vi "Filters_good_test.vi"() -> ()   [LabVIEW 2009]
uses:
  <vilib>/vision/NI_Vision_Development_Module.lvlib
panel:
  in  "Hough Skip":i32=1
  in  "LineFilterSelect":bool
  out "Hough Intensity Graph":i32[][](graph)
  out "Angle 2":i32
  out "X Intercept 2":i32
  in  "movement_limit":i32
  in  "check_block_size/2":i32
  in  "Waypoint Select":enum32{"Centroid", "Walk", "Mean Hough"}(radio)
  out "AverageTime (s)":dbl
  out "AverageTime (ms)":dbl
  out "ElapsedTime":u32
  out "Waypoint":cluster{i32, i32}
  in  "WP_DisplaySize/2":i32
  out "Filter Binary 2":T1(plugin-control)
  out "Filter Binary":T1(plugin-control)
  in  "file (use dialog)":path=path "C:/Documents and Settings/dgrieneisen/My Documents/Robotics/Athena/weights.fl"
  in  "Stop":bool
  in  "Filter Select":T2(radio)
  out "Filter Settings":T2(tab)
  in  "Red Range":cluster{"Lower value":i32, "Upper value":i32}={"Lower value"=120, "Upper value"=200}
  in  "Green Range":cluster{"Lower value":i32, "Upper value":i32}={"Lower value"=0, "Upper value"=255}
  in  "Blue Range":cluster{"Lower value":i32, "Upper value":i32}={"Lower value"=100, "Upper value"=255}
  in  "Color Mode":u16(ring) items=["RGB", "HSL", "HSV", "HSI"]
  in  "Hue Range":cluster{"Lower value":i32, "Upper value":i32}={"Lower value"=0, "Upper value"=255}
  in  "Saturation Range":cluster{"Lower value":i32, "Upper value":i32}={"Lower value"=0, "Upper value"=255}
  in  "Luma Range":cluster{"Lower value":i32, "Upper value":i32}={"Lower value"=0, "Upper value"=255}
  in  "Color Mode HSL":u16(ring)=1 items=["RGB", "HSL", "HSV", "HSI"]
  in  "Red Scalar":sgl=3.0
  in  "Green Scalar":sgl=3.0
  in  "Blue Scalar":sgl=3.3
  in  "Luma Scalar Low":sgl=4.0
  in  "Sat Scalar":sgl=2.5
  in  "Hue Scalar":sgl=5.0
  in  "Luma Scalar High":sgl=4.0
  in  "res/2":i32=3
  in  "Sample Rate":i32=3
  in  "ANN Level":dbl=0.5
  in  "ANN Out Switch":bool
  in  "Input Image Path":path=path "C:/Documents and Settings/dgrieneisen/My Documents/Robotics/Athena/image2004.jpg"
  out "'input Image":T1(plugin-control)
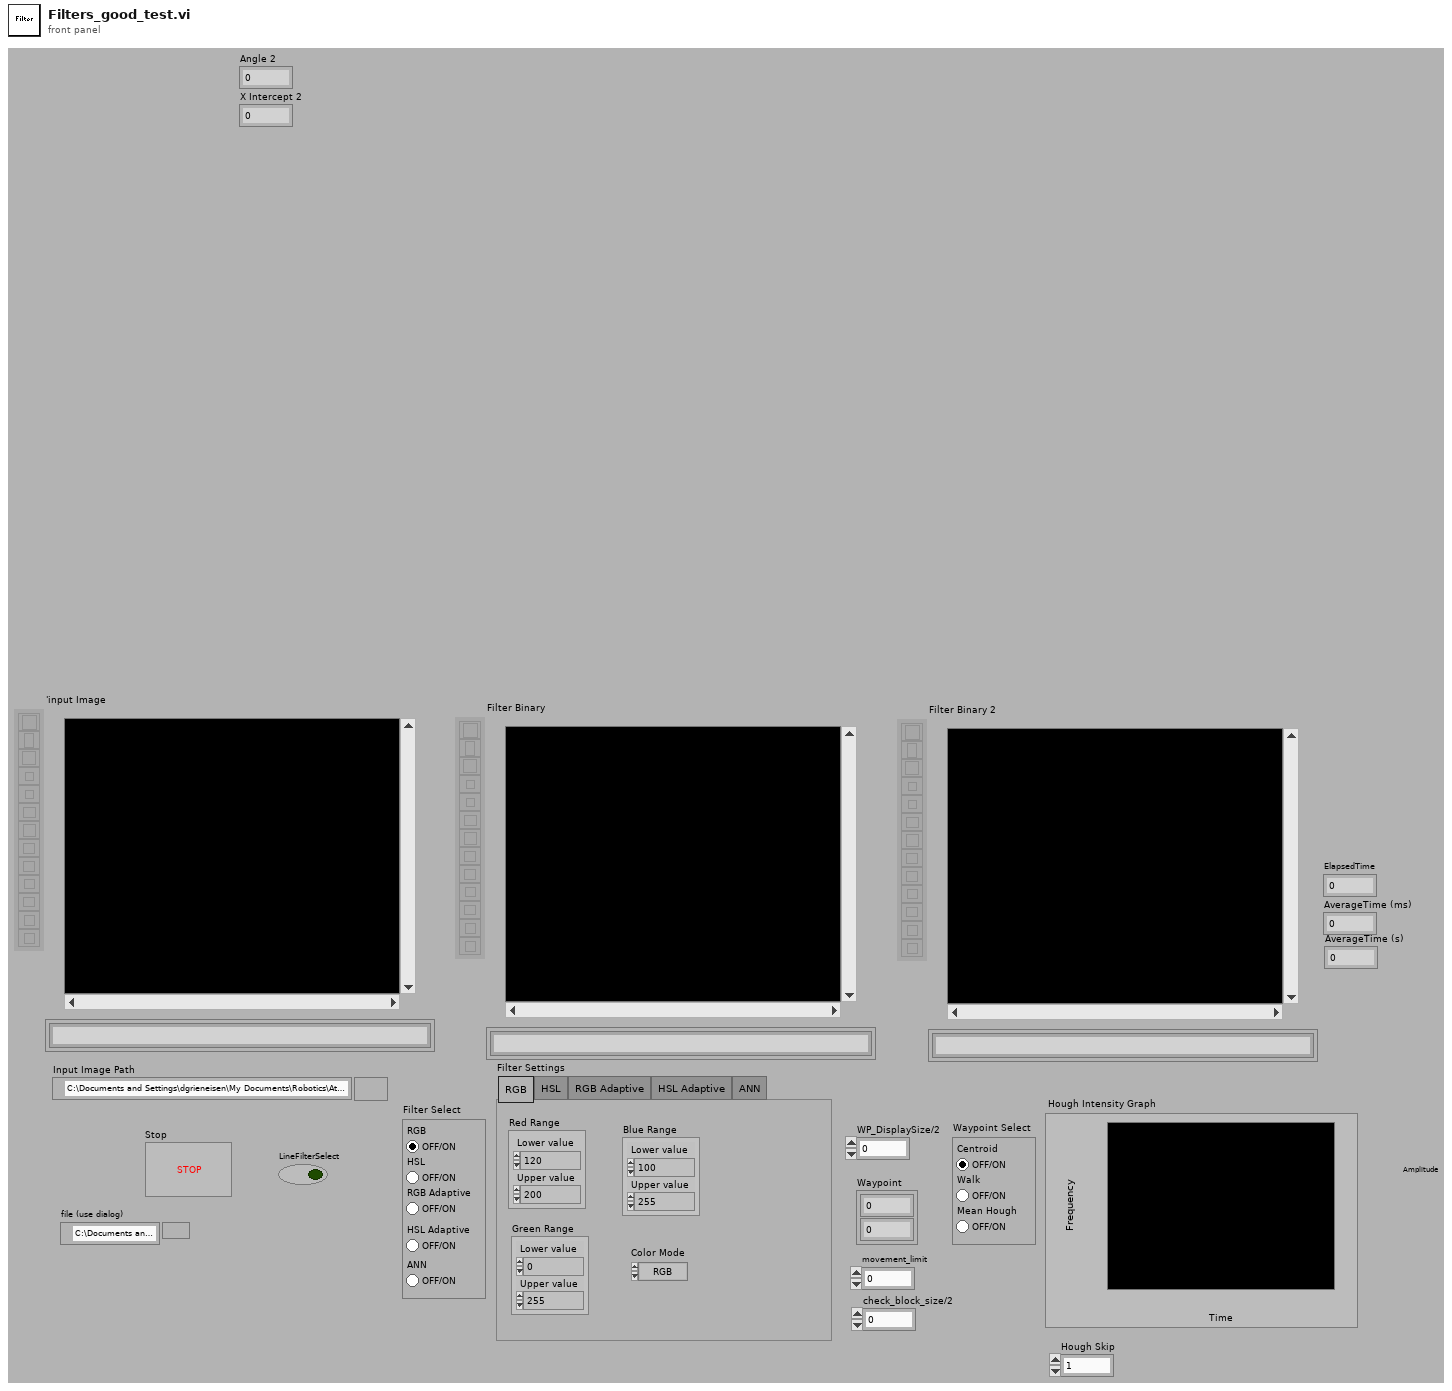
[diagram p1: front panel]
types:
  T1 = typedef "IMAQ Image.ctl" = refnum<image>
  T2 = enum32{"RGB", "HSL", "RGB Adaptive", "HSL Adaptive", "ANN"}
  T3 = typedef "Image Type" = u32
  T4 = cluster{"Num Hidden Layer":i32, "Function Final Layer":u16, "Function Hidden Layer":u16, dbl[], dbl[][]}
  T5 = cluster{"Left":i32, "Top":i32, "Right":i32, "Bottom":i32}
  T6 = cluster{"histogram":u32[], "Minimal Value":sgl, "Maximal Value":sgl, "Starting Value":sgl, "Interval Width":sgl, "Mean Value":sgl, "Standard  Variation":sgl, "Area (pixels)":i32}
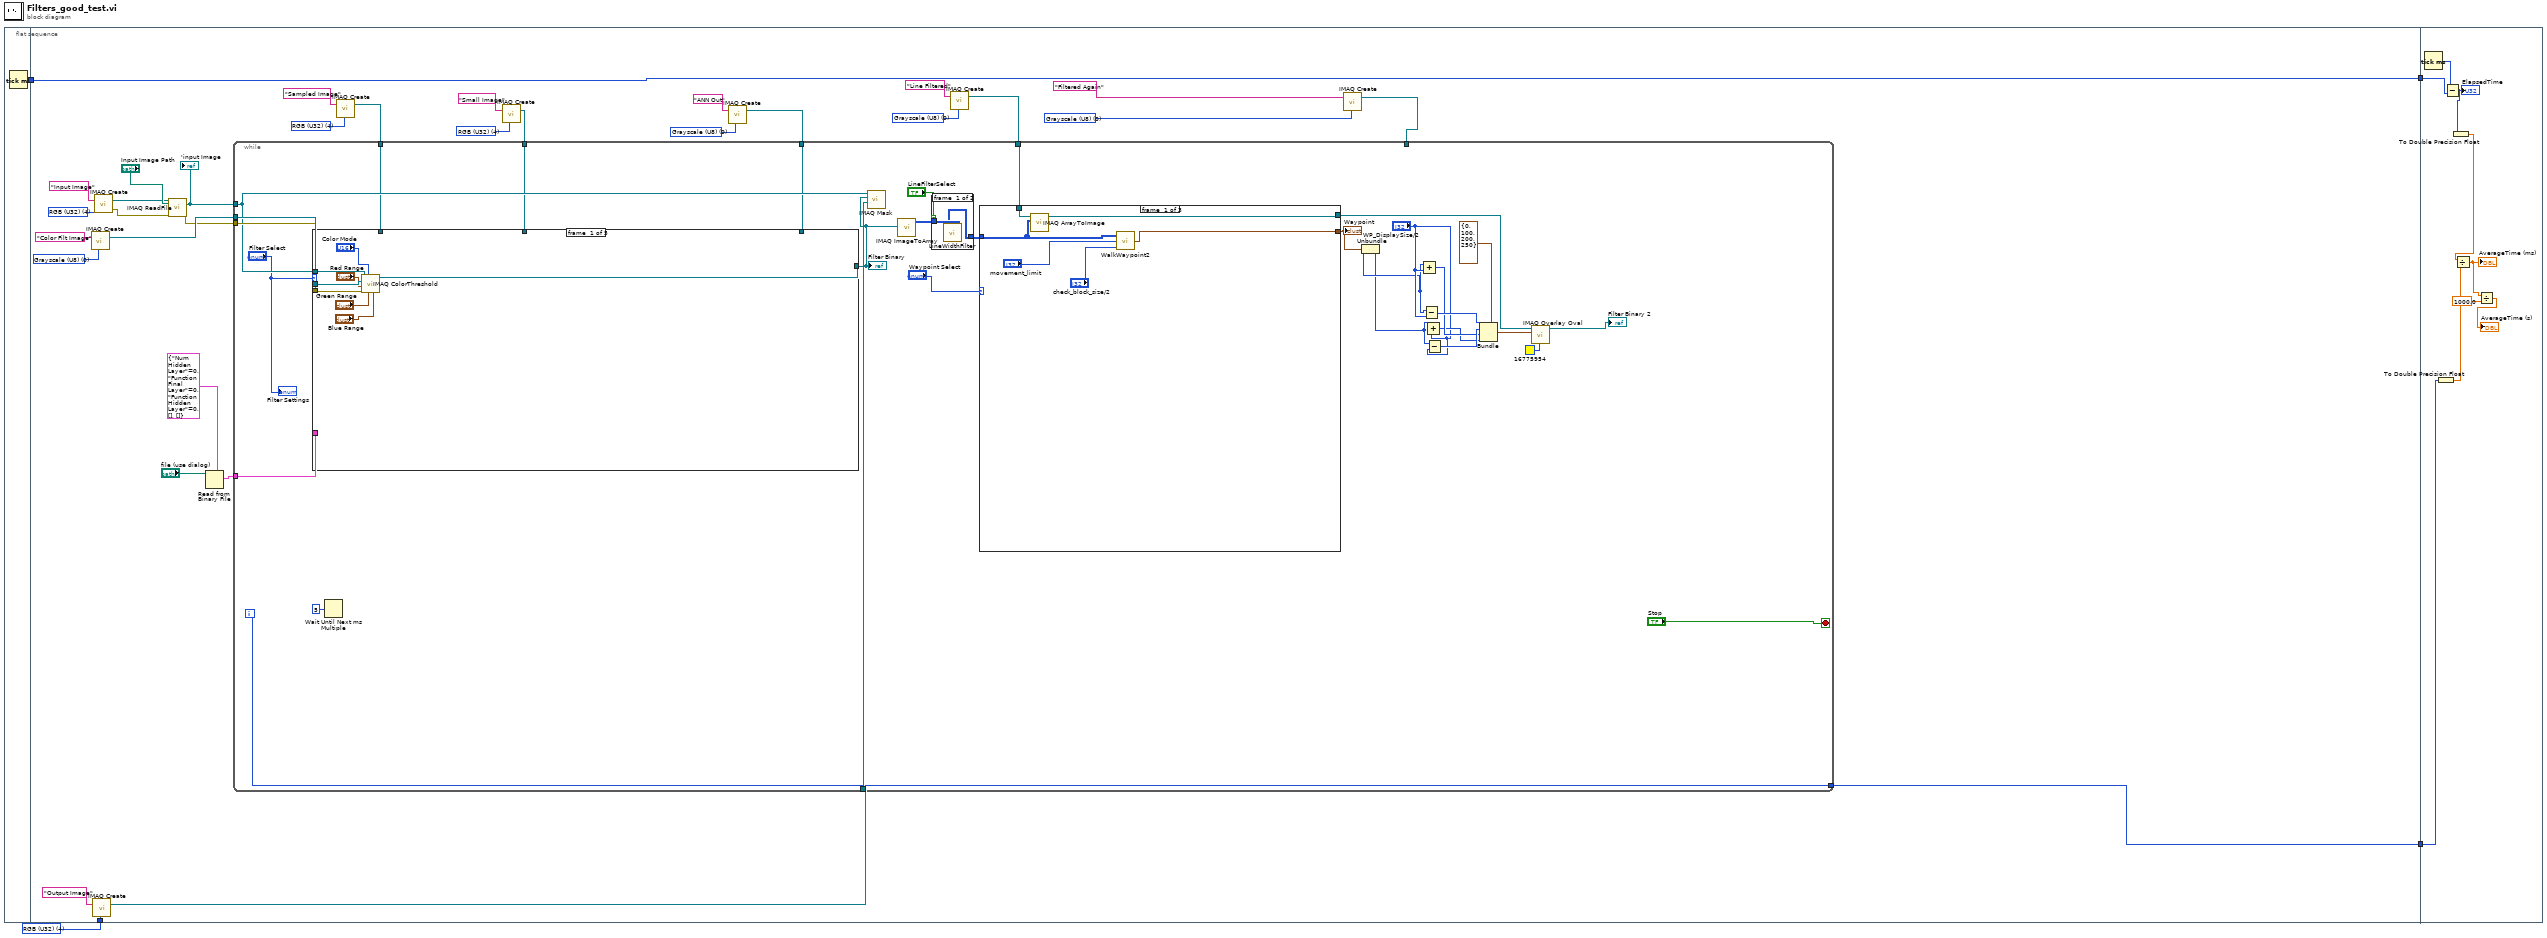
[diagram p0: block diagram]
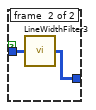
[diagram p2: hidden frame]
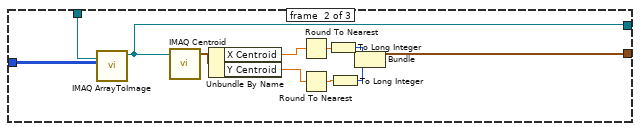
[diagram p3: hidden frame]
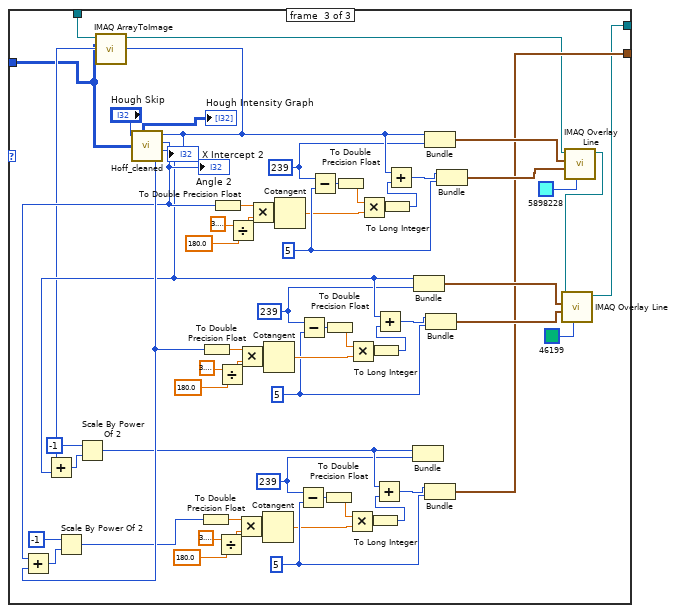
[diagram p4: hidden frame]
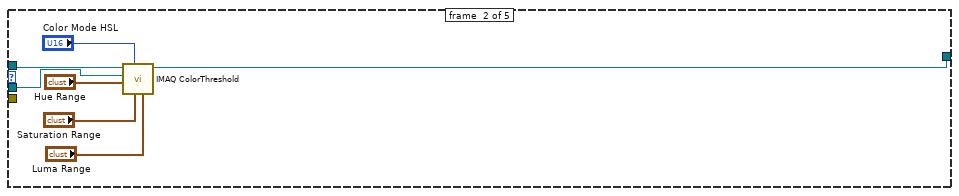
[diagram p5: hidden frame]
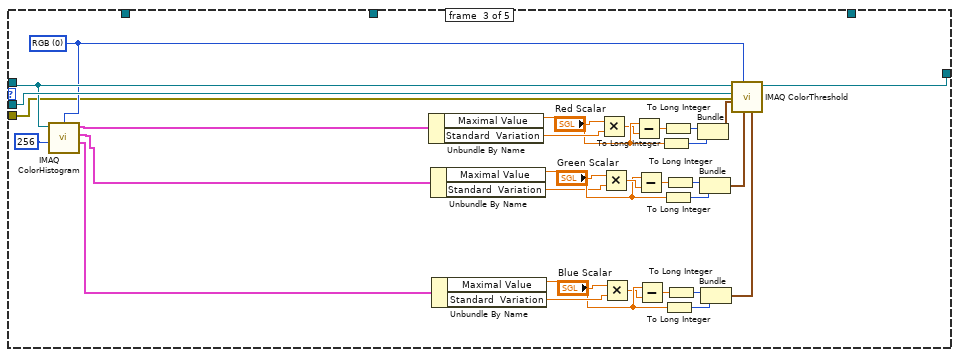
[diagram p6: hidden frame]
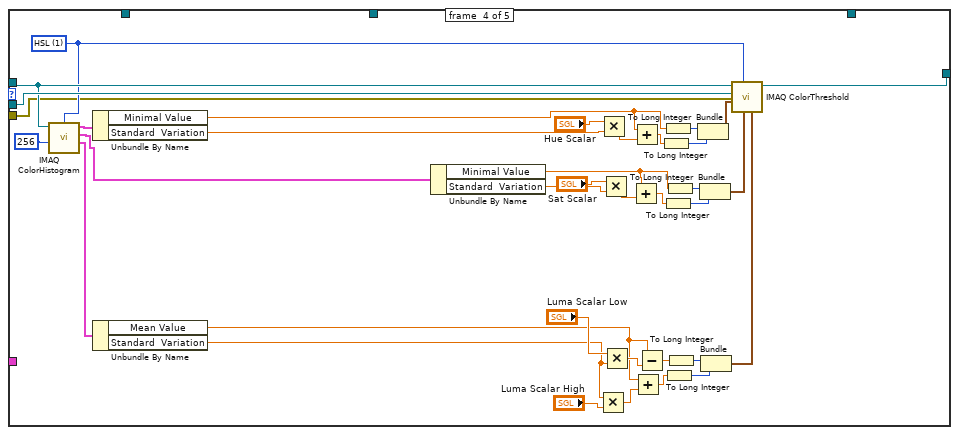
[diagram p7: hidden frame]
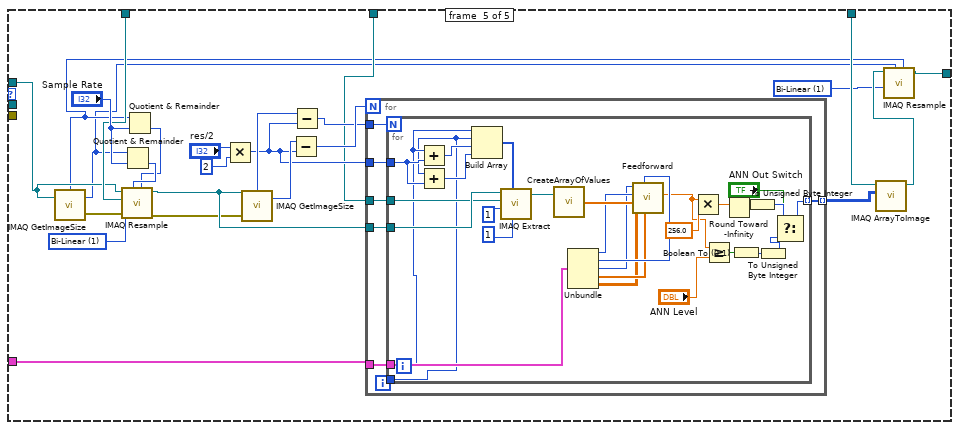
[diagram p8: hidden frame]
diagram:
  w4 = T3 4 items=["Grayscale (U8)", "Grayscale (I16)", "Grayscale (SGL)", "Complex (CSG)", "RGB (U32)", "HSL (U32)", "RGB (U64)", "Grayscale (U16)"] ("Image Type")
  n1 = flat-sequence {
    tunnel: [w5] -> w3
    tunnel: w4 -> [w34]
    tunnel: w3 -> [w8]
    tunnel: [w8] -> w2
    tunnel: [w7] -> w1
    tunnel: w2 -> [w306]
    tunnel: w1 -> [w305]
    frame #0 {
      n2 = Tick Count (ms)() -> (millisecond timer value=w5:u32)
    }
    frame #1 {
      w11 = T3 0 items=["Grayscale (U8)", "Grayscale (I16)", "Grayscale (SGL)", "Complex (CSG)", "RGB (U32)", "HSL (U32)", "RGB (U64)", "Grayscale (U16)"] ("Image Type")
      w12 = T3 0 items=["Grayscale (U8)", "Grayscale (I16)", "Grayscale (SGL)", "Complex (CSG)", "RGB (U32)", "HSL (U32)", "RGB (U64)", "Grayscale (U16)"] ("Image Type")
      w17 = T3 0 items=["Grayscale (U8)", "Grayscale (I16)", "Grayscale (SGL)", "Complex (CSG)", "RGB (U32)", "HSL (U32)", "RGB (U64)", "Grayscale (U16)"] ("Image Type")
      w21 = T3 4 items=["Grayscale (U8)", "Grayscale (I16)", "Grayscale (SGL)", "Complex (CSG)", "RGB (U32)", "HSL (U32)", "RGB (U64)", "Grayscale (U16)"] ("Image Type")
      w25 = T3 4 items=["Grayscale (U8)", "Grayscale (I16)", "Grayscale (SGL)", "Complex (CSG)", "RGB (U32)", "HSL (U32)", "RGB (U64)", "Grayscale (U16)"] ("Image Type")
      w36 = T3 0 items=["Grayscale (U8)", "Grayscale (I16)", "Grayscale (SGL)", "Complex (CSG)", "RGB (U32)", "HSL (U32)", "RGB (U64)", "Grayscale (U16)"] ("Image Type")
      w38 = T3 4 items=["Grayscale (U8)", "Grayscale (I16)", "Grayscale (SGL)", "Complex (CSG)", "RGB (U32)", "HSL (U32)", "RGB (U64)", "Grayscale (U16)"] ("Image Type")
      n3 = call "IMAQ Create"("Image Name"="Color Filt Image", "Image Type"=w36) -> ("New Image"=w30:T1)  [unwired: 2 in, 2 out]
      n4 = call "IMAQ Create"("Image Name"="Output Image", "Image Type"=w34) -> ("New Image"=w28:T1)  [unwired: 2 in, 2 out]
      n5 = call "IMAQ Create"("Image Name"="Input Image", "Image Type"=w38) -> ("New Image"=w27:T1, "error out"=w31:errorcluster)  [unwired: 2 in, 1 out]
      n6 = call "IMAQ ReadFile"("File Path"="Input Image Path", "error in (no error)"=w31, "Image"=w27) -> ("error out"=w29:errorcluster, "Image Out"=w26:T1)  [unwired: 4 in, 3 out]
      "'input Image" <- w26
      n7 = Read from Binary File(5:T4 {"Num Hidden Layer"=0, "Function Final Layer"=0, "Function Hidden Layer"=0, [], []} ("Cluster"), 11:"file (use dialog)") -> (2:w19:T4)  [unwired: 4 in, 3 out]
      n8 = call "IMAQ Create"("Image Name"="Sampled Image", "Image Type"=w25) -> ("New Image"=w23:T1)  [unwired: 2 in, 2 out]
      n9 = call "IMAQ Create"("Image Name"="Small Image", "Image Type"=w21) -> ("New Image"=w20:T1)  [unwired: 2 in, 2 out]
      n10 = call "IMAQ Create"("Image Name"="ANN Out", "Image Type"=w17) -> ("New Image"=w15:T1)  [unwired: 2 in, 2 out]
      n11 = call "IMAQ Create"("Image Name"="Line Filtered", "Image Type"=w12) -> ("New Image"=w6:T1)  [unwired: 2 in, 2 out]
      n12 = call "IMAQ Create"("Image Name"="Filtered Again", "Image Type"=w11) -> ("New Image"=w9:T1)  [unwired: 2 in, 2 out]
      n13 = while {
        tunnel: w30 -> [w69]
        tunnel: w29 -> [w68]
        tunnel: w28 -> [w67]
        tunnel: w26 -> [w66]
        tunnel: w23 -> [w63]
        tunnel: w20 -> [w62]
        tunnel: w19 -> [w61]
        tunnel: w15 -> [w60]
        tunnel: w6 -> [w57]
        tunnel: w9 -> [_]
        tunnel: [w48] -> w7
        i -> [w48]
        stop <- "Stop" stop-if-true
        n14 = case shown="\"ANN\"" "Filter Select" {
          tunnel: w69 -> [w161 w166 w200 w236 _]
          tunnel: w68 -> [w160 _ w187 w226 _]
          tunnel: w66 -> [w156 w167 w199 w235 w246]
          tunnel: [w154 w162 w201 w237 w241] -> w59
          tunnel: w63 -> [_ _ _ _ w247]
          tunnel: w62 -> [_ _ _ _ w245]
          tunnel: w61 -> [_ _ _ _ w244]
          tunnel: w60 -> [_ _ _ _ w243]
          frame #0 {
            n15 = call "IMAQ ColorThreshold"("Blue or Luma or Val or Inten Range"="Blue Range", "Green or Sat Range"="Green Range", "Color Mode"="Color Mode", "error in (no error)"=w160, "Red or Hue Range"="Red Range", "Image Dst"=w161, "Image Src"=w156) -> ("Image Dst Out"=w154:T1)  [unwired: 3 in, 1 out]
          }
          frame #1 {
            n16 = call "IMAQ ColorThreshold"("Blue or Luma or Val or Inten Range"="Luma Range", "Green or Sat Range"="Saturation Range", "Color Mode"="Color Mode HSL", "Red or Hue Range"="Hue Range", "Image Dst"=w166, "Image Src"=w167) -> ("Image Dst Out"=w162:T1)  [unwired: 4 in, 1 out]
          }
          frame #2 {
            w197 = u16 0 items=["RGB", "HSL", "HSV", "HSI"] ("Color Mode")
            n17 = call "IMAQ ColorHistogram"("Color Mode"=w197, "Image Src"=w199, "Number of Classes"=256) -> ("Red or Hue or X or L* Histogram Report"=w196:T6, "Green or Sat or Y or a* Histogram Report"=w170:T6, "Blue or Luma or Val or Inten or Z or b* Histogram Report"=w169:T6)  [unwired: 3 in, 1 out]
            n18 = Unbundle By Name(w196) -> ("Maximal Value"=w190:sgl, "Standard  Variation"=w192:sgl)
            n19 = Unbundle By Name(w170) -> ("Maximal Value"=w184:sgl, "Standard  Variation"=w182:sgl)
            n20 = Unbundle By Name(w169) -> ("Maximal Value"=w175:sgl, "Standard  Variation"=w177:sgl)
            n21 = Multiply(x="Red Scalar", y=w192) -> (x*y=w189:sgl)
            n22 = Multiply(x="Green Scalar", y=w182) -> (x*y=w185:sgl)
            n23 = Multiply(x="Blue Scalar", y=w177) -> (x*y=w174:sgl)
            n24 = Subtract(x=w190, y=w189) -> (x-y=w191:sgl)
            n25 = Subtract(x=w184, y=w185) -> (x-y=w183:sgl)
            n26 = Subtract(x=w175, y=w174) -> (x-y=w176:sgl)
            n27 = To Long Integer(number=w190) -> (32bit integer=w193:i32)
            n28 = To Long Integer(number=w191) -> (32bit integer=w194:i32)
            n29 = To Long Integer(number=w184) -> (32bit integer=w181:i32)
            n30 = To Long Integer(number=w175) -> (32bit integer=w178:i32)
            n31 = To Long Integer(number=w183) -> (32bit integer=w180:i32)
            n32 = To Long Integer(number=w176) -> (32bit integer=w179:i32)
            n33 = Bundle(w194, w193) -> (w195:cluster{i32, i32})  [unwired: 1 in]
            n34 = Bundle(w180, w181) -> (w172:cluster{i32, i32})  [unwired: 1 in]
            n35 = Bundle(w179, w178) -> (w171:cluster{i32, i32})  [unwired: 1 in]
            n36 = call "IMAQ ColorThreshold"("Blue or Luma or Val or Inten Range"=w171, "Green or Sat Range"=w172, "Color Mode"=w197, "error in (no error)"=w187, "Red or Hue Range"=w195, "Image Dst"=w200, "Image Src"=w199) -> ("Image Dst Out"=w201:T1)  [unwired: 3 in, 1 out]
          }
          frame #3 {
            w233 = u16 1 items=["RGB", "HSL", "HSV", "HSI"] ("Color Mode")
            n37 = call "IMAQ ColorHistogram"("Color Mode"=w233, "Image Src"=w235, "Number of Classes"=256) -> ("Red or Hue or X or L* Histogram Report"=w232:T6, "Green or Sat or Y or a* Histogram Report"=w216:T6, "Blue or Luma or Val or Inten or Z or b* Histogram Report"=w215:T6)  [unwired: 3 in, 1 out]
            n38 = Unbundle By Name(w232) -> ("Minimal Value"=w213:sgl, "Standard  Variation"=w228:sgl)
            n39 = Unbundle By Name(w215) -> ("Mean Value"=w203:sgl, "Standard  Variation"=w206:sgl)
            n40 = Unbundle By Name(w216) -> ("Minimal Value"=w211:sgl, "Standard  Variation"=w224:sgl)
            n41 = Multiply(x=w206, y="Luma Scalar High") -> (x*y=w204:sgl)
            n42 = Multiply(x="Hue Scalar", y=w228) -> (x*y=w214:sgl)
            n43 = Multiply(x="Sat Scalar", y=w224) -> (x*y=w210:sgl)
            n44 = Multiply(x="Luma Scalar Low", y=w206) -> (x*y=w219:sgl)
            n45 = Add(x=w211, y=w210) -> (x+y=w209:sgl)
            n46 = Add(x=w213, y=w214) -> (x+y=w212:sgl)
            n47 = Add(x=w203, y=w204) -> (x+y=w205:sgl)
            n48 = Subtract(x=w203, y=w219) -> (x-y=w220:sgl)
            n49 = To Long Integer(number=w212) -> (32bit integer=w229:i32)
            n50 = To Long Integer(number=w213) -> (32bit integer=w230:i32)
            n51 = To Long Integer(number=w209) -> (32bit integer=w223:i32)
            n52 = To Long Integer(number=w205) -> (32bit integer=w202:i32)
            n53 = To Long Integer(number=w211) -> (32bit integer=w222:i32)
            n54 = To Long Integer(number=w220) -> (32bit integer=w221:i32)
            n55 = Bundle(w230, w229) -> (w231:cluster{i32, i32})  [unwired: 1 in]
            n56 = Bundle(w222, w223) -> (w218:cluster{i32, i32})  [unwired: 1 in]
            n57 = Bundle(w221, w202) -> (w217:cluster{i32, i32})  [unwired: 1 in]
            n58 = call "IMAQ ColorThreshold"("Blue or Luma or Val or Inten Range"=w217, "Green or Sat Range"=w218, "Color Mode"=w233, "error in (no error)"=w226, "Red or Hue Range"=w231, "Image Dst"=w236, "Image Src"=w235) -> ("Image Dst Out"=w237:T1)  [unwired: 3 in, 1 out]
          }
          frame #4 {
            w240 = u32 1 items=["Zero Order", "Bi-Linear", "Quadratic", "Cubic Spline"] ("Interpolation Type")
            w258 = u32 1 items=["Zero Order", "Bi-Linear", "Quadratic", "Cubic Spline"] ("Interpolation Type")
            n59 = call "IMAQ GetImageSize"("Image"=w246) -> ("Y Resolution"=w238:i32, "X Resolution"=w239:i32, "error out"=w262:errorcluster)  [unwired: 3 in]
            n60 = Quotient & Remainder(x=w238, y="Sample Rate") -> (floor(x/y)=w261:i32)  [unwired: 1 out]
            n61 = Quotient & Remainder(x=w239, y="Sample Rate") -> (floor(x/y)=w260:i32)  [unwired: 1 out]
            n62 = call "IMAQ Resample"("X Resolution"=w260, "Y Resolution"=w261, "error in (no error)"=w262, "Interpolation Type"=w258, "Image Dst"=w247, "Image Src"=w246) -> ("error out"=w248:errorcluster, "Image Dst Out"=w252:T1)  [unwired: 4 in]
            n63 = Multiply(x="res/2", y=2) -> (x*y=w253:i32)
            n64 = call "IMAQ GetImageSize"("Image"=w252, "error in (no error)"=w248) -> ("Y Resolution"=w257:i32, "X Resolution"=w254:i32)  [unwired: 2 in, 1 out]
            n65 = Subtract(x=w257, y=w253) -> (x-y=w250:i32)
            n66 = Subtract(x=w254, y=w253) -> (x-y=w249:i32)
            n67 = for {
              N: w250 -> [_]
              tunnel: w253 -> [w269]
              tunnel: w252 -> [w268]
              tunnel: w244 -> [w267]
              tunnel: [w266] -> w251 mode=indexing
              tunnel: w245 -> [w265]
              tunnel: w249 -> [w264]
              i -> [w263]
              n68 = for {
                N: w264 -> [_]
                tunnel: w269 -> [w295]
                tunnel: w268 -> [w293]
                tunnel: w267 -> [w290]
                tunnel: [w271] -> w266 mode=indexing
                tunnel: w265 -> [w284]
                tunnel: w263 -> [w280]
                i -> [w281]
                n69 = Add(x=w281, y=w295) -> (x+y=w297:i32)
                n70 = Add(x=w280, y=w295) -> (x+y=w296:i32)
                n71 = Build Array(w281, w280, w297, w296) -> (w294:i32[])
                n72 = call "IMAQ Extract"("Y Step Size"=1, "Optional Rectangle"=w294, "X Step Size"=1, "Image Dst"=w284, "Image Src"=w293) -> ("Image Dst Out"=w292:T1)  [unwired: 1 in, 5 out]
                n73 = call "CreateArrayOfValues.vi"("Image Out"=w292) -> ("Array"=w291:dbl[])  [unwired: 1 in]
                n74 = Unbundle(w290) -> ("Num Hidden Layer"=w289:i32, "Function Final Layer"=w288:u16, "Function Hidden Layer"=w287:u16, w286:dbl[], w285:dbl[][])
                n75 = call "Feedforward.vi"("Final Weights"=w286, "Function Final Layer"=w288, "Hidden Weights"=w285, "Inputs"=w291, "Num Hidden Layer"=w289, "Function Hidden Layer"=w287) -> ("Output"=w276:dbl)  [unwired: 3 out]
                n76 = Multiply(x=w276, y=256.0) -> (x*y=w282:dbl)
                n77 = Greater Or Equal?(x=w276, y="ANN Level") -> (x >= y?=w278:bool)
                n78 = Round Toward -Infinity(1:w282) -> (0:w275:dbl)
                n79 = Boolean To (0,1)(Boolean=w278) -> (0, 1=w274:i16)
                n80 = To Unsigned Byte Integer(number=w275) -> (unsigned 8bit integer=w272:u8)
                n81 = To Unsigned Byte Integer(number=w274) -> (unsigned 8bit integer=w273:u8)
                n82 = Select(t=w272, s="ANN Out Switch", f=w273) -> (s? t:f=w271:u8)
              }
            }
            n83 = call "IMAQ ArrayToImage"("Image Pixels (U8)"=w251, "Image"=w243) -> ("Image Out"=w242:T1)  [unwired: 8 in, 1 out]
            n84 = call "IMAQ Resample"("X Resolution"=w239, "Y Resolution"=w238, "Interpolation Type"=w240, "Image Src"=w242) -> ("Image Dst Out"=w241:T1)  [unwired: 6 in, 1 out]
          }
        }
        "Filter Binary" <- w59
        n85 = Wait Until Next ms Multiple(millisecond multiple=u32 5) -> ()  [unwired: 1 out]
        n86 = call "IMAQ Mask"("Image Dst"=w67, "Image Mask"=w59, "Image Src"=w66) -> ()  [unwired: 2 in, 2 out]
        n87 = call "IMAQ ImageToArray"("Image"=w59) -> ("Image Pixels (U8)"=w58:u8[][])  [unwired: 3 in, 4 out]
        n88 = case shown="False" "LineFilterSelect" {
          tunnel: w58 -> [w71 w73]
          tunnel: [w70 w72] -> w40
          frame #0 {
            n89 = call "LineWidthFilter.vi"("Image Pixels (U8) 2"=w71) -> ("Image Pixels (U8)"=w70:u8[][])
          }
          frame #1 {
            n90 = call "LineWidthFilter3.vi"("Image Pixels (U8) 2"=w73) -> ("Image Pixels (U8)"=w72:u8[][])
          }
        }
        n91 = case shown="\"Mean Hough\"" "Waypoint Select" {
          tunnel: w57 -> [w76 w90 w94]
          tunnel: [w77 w80 w96] -> w43
          tunnel: w40 -> [w75 w89 w95]
          tunnel: [w74 w88 w92] -> w47
          frame #0 {
            n92 = call "IMAQ ArrayToImage"("Image Pixels (U8)"=w75, "Image"=w76) -> ("Image Out"=w74:T1)  [unwired: 8 in, 1 out]
            n93 = call "WalkWaypoint2.vi"("check_block_size/2"="check_block_size/2", "movement_limit"="movement_limit", "Image Pixels (U8)"=w75) -> ("WaypointOut"=w77:cluster{i32, i32})
          }
          frame #1 {
            n94 = call "IMAQ ArrayToImage"("Image Pixels (U8)"=w89, "Image"=w90) -> ("Image Out"=w88:T1)  [unwired: 8 in, 1 out]
            n95 = call "IMAQ Centroid"("Image"=w88) -> ("Centroid"=w87:cluster{"X Centroid":sgl, "Y Centroid":sgl})  [unwired: 3 in, 1 out]
            n96 = Unbundle By Name(w87) -> ("X Centroid"=w84:sgl, "Y Centroid"=w83:sgl)
            n97 = Round To Nearest(number=w84) -> (nearest integer value=w86:sgl)
            n98 = Round To Nearest(number=w83) -> (nearest integer value=w85:sgl)
            n99 = To Long Integer(number=w86) -> (32bit integer=w82:i32)
            n100 = To Long Integer(number=w85) -> (32bit integer=w81:i32)
            n101 = Bundle(w82, w81) -> (w80:cluster{i32, i32})  [unwired: 1 in]
          }
          frame #2 {
            w139 = 5 ("y")
            w138 = 239 ("y")
            w117 = 5 ("y")
            w118 = 239 ("y")
            w106 = 5 ("y")
            w105 = 239 ("y")
            n102 = call "IMAQ ArrayToImage"("Image Pixels (U8)"=w95, "Image"=w94) -> ("Image Out"=w93:T1)  [unwired: 8 in, 1 out]
            n103 = call "Hoff_cleaned.vi"("Skip-1"="Hough Skip", "Image Pixels (U8)"=w95) -> ("3 times averaged"=→"Hough Intensity Graph":i32[][], "X Intercept"=w150:i32, "Angle"=w152:i32, "X Intercept 2"=w151:i32, "Angle 2"=w153:i32)  [unwired: 2 in]
            "Angle 2" <- w152
            "X Intercept 2" <- w150
            n104 = Add(x=w152, y=w153) -> (x+y=w149:i32)
            n105 = Add(x=w150, y=w151) -> (x+y=w148:i32)
            n106 = Scale By Power Of 2(n=i16 -1, x=w149) -> (x*2^n=w145:i32)
            n107 = Scale By Power Of 2(n=i16 -1, x=w148) -> (x*2^n=w147:i32)
            n108 = To Double Precision Float(number=w145) -> (double precision float=w133:dbl)
            n109 = To Double Precision Float(number=w153) -> (double precision float=w123:dbl)
            n110 = To Double Precision Float(number=w152) -> (double precision float=w100:dbl)
            n111 = Divide(x=3.141592653589793, y=180.0) -> (x/y=w134:dbl)
            n112 = Divide(x=3.141592653589793, y=180.0) -> (x/y=w122:dbl)
            n113 = Divide(x=3.141592653589793, y=180.0) -> (x/y=w101:dbl)
            n114 = Multiply(x=w133, y=w134) -> (x*y=w135:dbl)
            n115 = Multiply(x=w123, y=w122) -> (x*y=w121:dbl)
            n116 = Multiply(x=w100, y=w101) -> (x*y=w102:dbl)
            n117 = Cotangent(1:w135) -> (0:w136:dbl)
            n118 = Cotangent(1:w121) -> (0:w120:dbl)
            n119 = Cotangent(1:w102) -> (0:w103:dbl)
            n120 = Subtract(x=w138, y=w139) -> (x-y=w140:i32)
            n121 = Subtract(x=w118, y=w117) -> (x-y=w116:i32)
            n122 = Subtract(x=w105, y=w106) -> (x-y=w109:i32)
            n123 = To Double Precision Float(number=w140) -> (double precision float=w141:dbl)
            n124 = To Double Precision Float(number=w116) -> (double precision float=w115:dbl)
            n125 = To Double Precision Float(number=w109) -> (double precision float=w110:dbl)
            n126 = Multiply(x=w141, y=w136) -> (x*y=w142:dbl)
            n127 = Multiply(x=w115, y=w120) -> (x*y=w114:dbl)
            n128 = Multiply(x=w110, y=w103) -> (x*y=w111:dbl)
            n129 = To Long Integer(number=w142) -> (32bit integer=w143:i32)
            n130 = To Long Integer(number=w114) -> (32bit integer=w113:i32)
            n131 = Add(x=w147, y=w143) -> (x+y=w137:i32)
            n132 = Add(x=w151, y=w113) -> (x+y=w119:i32)
            n133 = To Long Integer(number=w111) -> (32bit integer=w112:i32)
            n134 = Add(x=w150, y=w112) -> (x+y=w104:i32)
            n135 = Bundle(w147, "y"=w138) -> ()  [unwired: 1 in, 1 out]
            n136 = Bundle("X Intercept 2"=w151, "y"=w118) -> (w128:cluster{"X Intercept 2":i32, "y":i32})  [unwired: 1 in]
            n137 = Bundle("X Intercept"=w150, "y"=w105) -> (w107:cluster{"X Intercept":i32, "y":i32})  [unwired: 1 in]
            n138 = Bundle(w137, "y"=w139) -> (w96:cluster{i32, "y":i32})  [unwired: 1 in]
            n139 = Bundle(w119, "y"=w117) -> (w129:cluster{i32, "y":i32})  [unwired: 1 in]
            n140 = Bundle(w104, "y"=w106) -> (w108:cluster{i32, "y":i32})  [unwired: 1 in]
            n141 = call "IMAQ Overlay Line"("Color"=u32 5898228, "End Point"=w108, "Start Point"=w107, "Image"=w93) -> ("Image Out"=w130:T1)  [unwired: 6 in, 1 out]
            n142 = call "IMAQ Overlay Line"("Color"=u32 46199, "End Point"=w129, "Start Point"=w128, "Image"=w130) -> ("Image Out"=w92:T1)  [unwired: 6 in, 1 out]
          }
        }
        "Waypoint" <- w43
        n143 = Unbundle(w43) -> (w46:i32, "y"=w45:i32)
        n144 = Add(x=w46, y="WP_DisplaySize/2") -> (x+y=w53:i32)
        n145 = Subtract(x=w46, y="WP_DisplaySize/2") -> (x-y=w55:i32)
        n146 = Add(x=w45, y="WP_DisplaySize/2") -> (x+y=w52:i32)
        n147 = Subtract(x=w45, y="WP_DisplaySize/2") -> (x-y=w54:i32)
        n148 = Bundle(cluster=T5 {"Left"=0, "Top"=100, "Right"=200, "Bottom"=250} ("Bounding Rectangle"), "Left"=w55, "Top"=w54, "Right"=w53, "Bottom"=w52) -> (w51:T5)
        n149 = call "IMAQ Overlay Oval"("Color"=u32 16775954, "Bounding Rectangle"=w51, "Image"=w47) -> ("Image Out"=→"Filter Binary 2":T1)  [unwired: 7 in, 1 out]
        "Filter Settings" <- "Filter Select"
      }
    }
    frame #2 {
      n150 = Tick Count (ms)() -> (millisecond timer value=w307:u32)
      n151 = To Double Precision Float(number=w305) -> (double precision float=w303:dbl)
      n152 = Subtract(x=w307, y=w306) -> (x-y=w304:u32)
      "ElapsedTime" <- w304
      n153 = To Double Precision Float(number=w304) -> (double precision float=w302:dbl)
      n154 = Divide(x=w302, y=w303) -> (x/y=w301:dbl)
      "AverageTime (ms)" <- w301
      n155 = Divide(x=w301, y=1000.0) -> (x/y=→"AverageTime (s)":dbl)
    }
  }
